vi "test tree.vi"() -> ()   [LabVIEW 2011]
uses:
  <userlib>/MSC-Tree/SW Code/Tree -string-/sub VIs/spring action.ctl
panel:
  in  "Tree":string(tree)
  in  "indentation":i32[](array[numeric])=[0, 1, 1, 2, 0]
  in  "symbols":i32[](array[numeric])=[0, 6, 14, 13, 28]
  in  "bg colors":u32[](array[colorbox])=[16777164, 13434879, 13434828, 16777226, 13816530]
  in  "fg colors":u32[](array[colorbox])=[0, 1442031, 16711680, 1985280, 0]
  in  "item strings":string[][](array[string])=[["a", "1"], ["a1", "2"], ["a2", "3"], ["b", "File"], ["b1", "DAQ"]]
  # "Error 16 = number of columns incorrect"
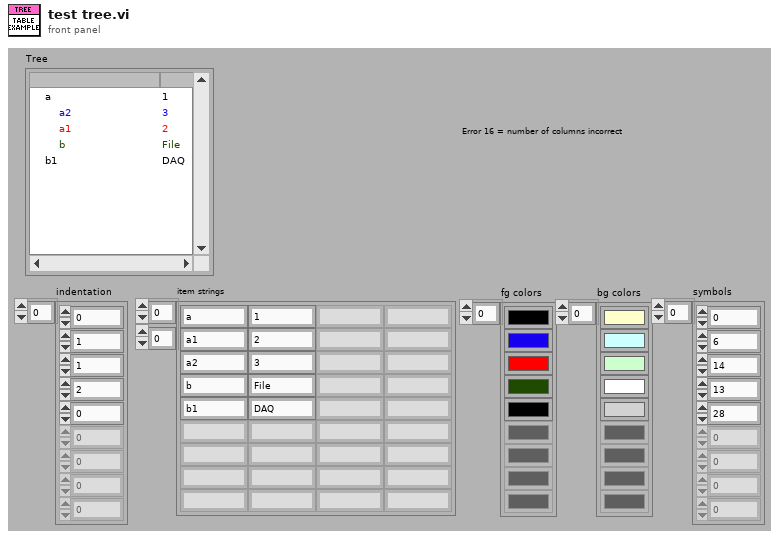
[diagram p1: front panel]
types:
  T1 = typedef "spring action.ctl" = enum16{"_init", "_add tree", "set itemstrings", "set fg colors", "set bg colors", "set symbols", "get tags", "get itemstrings", "get fg colors", "get bg colors", "get symbols", "empty tree", "update from tree"}
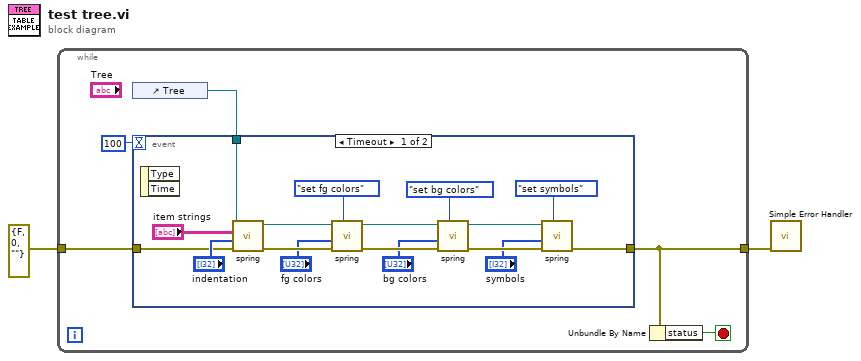
[diagram p0: block diagram]
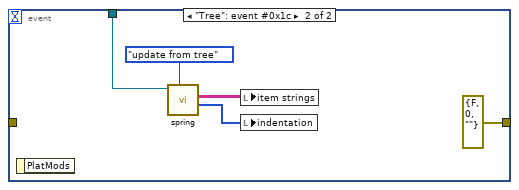
[diagram p2: hidden frame]
diagram:
  n1 = while {
    tunnel: errorcluster {"status"=FALSE, "code"=0, "source"=""} ("error out") -> [w4]
    tunnel: [w3] -> w1
    stop <- w5 stop-if-true
    n2 = control-ref of="Tree"() -> (w6:refnum<vi>)
    n3 = event shown="[0] Timeout" {
      selector: _ -> [_ _]
      dyn-events: _ -> [_ _]
      timeout: 100 -> [_ _]
      tunnel: w6 -> [w9 w28]
      tunnel: [w13 errorcluster {"status"=FALSE, "code"=0, "source"=""} ("error out")] -> w3
      tunnel: w4 -> [w12 _]
      event Timeout {
        n4 = event-data() -> ()  [unwired: 1 in, 2 out]
        n5 = call <userlib>:"spring.vi"("error in (no error)"=w12, "indentation/item symbols/colors in"="indentation", "item strings in"="item strings", "tree RefNum in"=w9) -> ("error out"=w20:errorcluster, "dup tree RefNum"=w11:refnum<vi>)  [unwired: 4 in, 2 out]
        n6 = call <userlib>:"spring.vi"("action (set itemstrings)"=spring_action."set fg colors" ("action (set)"), "error in (no error)"=w20, "indentation/item symbols/colors in"="fg colors", "tree RefNum in"=w11) -> ("error out"=w19:errorcluster, "dup tree RefNum"=w10:refnum<vi>)  [unwired: 4 in, 2 out]
        n7 = call <userlib>:"spring.vi"("action (set itemstrings)"=spring_action."set bg colors" ("action (set)"), "error in (no error)"=w19, "indentation/item symbols/colors in"="bg colors", "tree RefNum in"=w10) -> ("error out"=w18:errorcluster, "dup tree RefNum"=w8:refnum<vi>)  [unwired: 4 in, 2 out]
        n8 = call <userlib>:"spring.vi"("action (set itemstrings)"=spring_action."set symbols" ("action (set)"), "error in (no error)"=w18, "indentation/item symbols/colors in"="symbols", "tree RefNum in"=w8) -> ("error out"=w13:errorcluster)  [unwired: 4 in, 3 out]
      }
      event "Tree": event #0x1c {
        n9 = event-data() -> ()  [unwired: 1 in, 1 out]
        n10 = call <userlib>:"spring.vi"("action (set itemstrings)"=spring_action."update from tree" ("action (set)"), "tree RefNum in"=w28) -> ("item symbols/colors out"=w26:i32[], "item strings out"=w29:string[][])  [unwired: 6 in, 2 out]
        n11 = local write "item strings"(w29) -> ()
        n12 = local write "indentation"(w26) -> ()
      }
    }
    n13 = Unbundle By Name(w3) -> ("status"=w5:bool)
  }
  n14 = call <vilib>:"Simple Error Handler.vi"("error in (no error)"=w1) -> ()  [unwired: 4 in, 5 out]
